vi "Servo MSMT ET Create Delay Evals.vi"(8 "error in (no error)":errorcluster, 10 "Step In":refnum<k7>, 11 "Servo MSMT in":refnum<class "Servo MSMT.lvclass">) -> (0 "error out":errorcluster, 2 "Step Out":refnum<k7>, 3 "Servo MSMT out":refnum<class "Servo MSMT.lvclass">)   [LabVIEW 2018, in "Servo MSMT.lvlib" / "Servo MSMT.lvclass"]
uses:
  Servo MSMT.lvclass
  C:/Sequence Automation/Plugins/Measurement Interface.lvlibp/Measurement Interface.lvclass
  Plugins/Measurement Interface.lvlibp/Private Methods/Measurement Name/Read Measurement Name.vi
  Plugins/Measurement Interface.lvlibp/Private Methods/Engine Reference/Read Engine Reference.vi
  Plugins/Measurement Interface.lvlibp/Private Methods/Measurement Parameters/Read Measurement Parameters.vi
  Plugins/String Database.lvlibp/String Database.lvclass
  Plugins/SeqAuto Evaluations.lvlibp/ET Evaluations/ET_Delay_Sweep.lvclass
  Plugins/Test Number and Bin Generator.lvlibp/Test Number and Bin Generator/Test Number and Bin Generator.lvclass
  Plugins/TestStand API Tools (TSAT).lvlibp/Step Actions/TSAT Step Actions.lvlib
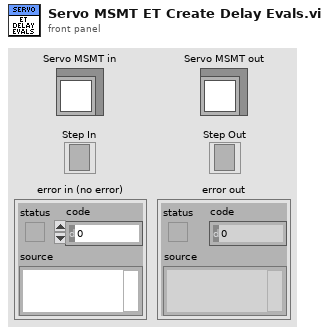
[diagram p1: front panel]
types:
  T1 = typedef "TestStand API Tools (TSAT).lvlibp/TSAT Evaluation Actions.lvlib/TSAT Evaluation.ctl" = cluster{"Test Name":string, "Pin":string, "Units":string, "SI Scaling":T2, "Test Number":i32, "Published Data Id":string, "Low Limit":dbl, "High Limit":dbl, "Export Data Location":string, "Software Bin":i64, "Evaluation Type":T3, "Test Data Source":string}
  T2 = typedef "TestStand API Tools (TSAT).lvlibp/TSAT Evaluation Actions.lvlib/TSAT Eval SI Unit Scaling.ctl" = i16
  T3 = typedef "TestStand API Tools (TSAT).lvlibp/TSAT Evaluation Actions.lvlib/TSAT Evaluation Type.ctl" = enum16{"Numeric Limit", "Pass/Fail", "None"}
  T4 = typedef "Test Number and Bin Generator.lvlibp/Test Number and Bin Generator.lvclass/Session Handle.ctl" = refnum<data-value>
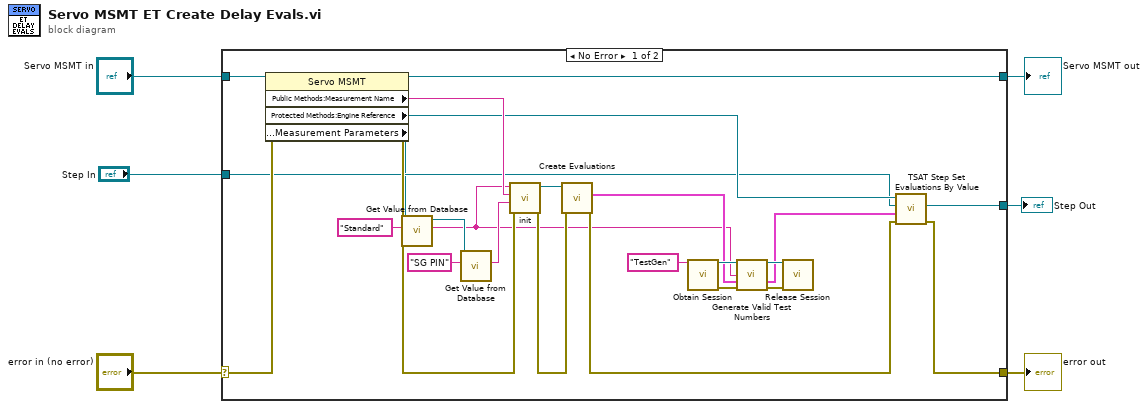
[diagram p0: block diagram]
diagram:
  n1 = case shown="No Error" "error in (no error)" {
    selector: "error in (no error)" -> [w31 w34]
    tunnel: [w16 w34] -> w5
    tunnel: [w29 w33] -> w3
    tunnel: "Servo MSMT in" -> [w30 w33]
    tunnel: "Step In" -> [w14 w32]
    tunnel: [w13 w32] -> w1
    frame No Error {
      n2 = property class="Servo MSMT"(reference=w30, error in=w31) -> (reference out=w29:refnum<class "Servo MSMT.lvclass">, error out=w27:errorcluster, "Public Methods:Measurement Name"=w28:string, "Protected Methods:Engine Reference"=w15:refnum<k7>, "Protected Methods:Measurement Parameters"=w12:refnum<class "String Database.lvclass">)
      n3 = call "Get Value from Database.vi"("Entry Name"="Standard", "Message in"=w12) -> ("Entry Value"=w7:string, "Message out"=w10:refnum<class "String Database.lvclass">)  [unwired: 6 in, 2 out]
      n4 = call "Get Value from Database.vi"("Entry Name"="SG PIN", "Message in"=w10) -> ("Entry Value"=w8:string)  [unwired: 6 in, 3 out]
      n5 = call "init.vi"("error in (no error)"=w27, "SG Pin"=w8, "Measurement Name"=w28, "Standard"=w7) -> ("error out"=w26:errorcluster, "ET_Delay_Sweep out"=w25:refnum<class "ET_Delay_Sweep.lvclass">)  [unwired: 6 in]
      n6 = call-dynamic "Create Evaluations.vi"("error in (no error)"=w26, "IEvaluation in"=w25) -> ("error out"=w17:errorcluster, "Evaluations Out"=w21:T1[])  [unwired: 7 in, 1 out]
      n7 = call "Obtain Session.vi"("Session  Name ()"="TestGen") -> ("Session Handle"=w23:T4, "error out"=w22:errorcluster)  [unwired: 13 in]
      n8 = call "Generate Valid Test Numbers.vi"("Session Handle in"=w23, "Test Group"=w7, "Evaluations In"=w21, "error in (no error)"=w22) -> ("Session Handle out"=w20:T4, "Evaluations Out"=w18:T1[], "error out"=w19:errorcluster)  [unwired: 9 in]
      n9 = call "Release Session.vi"("Session Handle"=w20, "error in (no error)"=w19) -> ()  [unwired: 13 in, 1 out]
      n10 = call "TSAT Step Set Evaluations By Value.vi"("Error In"=w17, "Evaluation Data"=w18, "Step In"=w14, "Engine In"=w15) -> ("Error Out"=w16:errorcluster, "Step Out"=w13:refnum<k7>)  [unwired: 5 in, 1 out]
    }
    frame Error {
    }
  }
  "error out" <- w5
  "Servo MSMT out" <- w3
  "Step Out" <- w1
